vi "Configure Serial Bus (UART - Basic).vi"(0 "VISA resource name":refnum<visa-resource-name>, 1 "Bit Order (0: LSB First)":i32(ring) items=["LSB First", "MSB First"], 2 "Parity (0: Even)":i32(ring) items=["Even", "Odd", "None"], 3 "Data Bits (5 bits)":i32=5, 5 "Serial Bus Name (1: Serial Bus 1)":i32(ring)=1 items=["Serial Bus 1"=1, "Serial Bus 2"=2], 7 "Decode Base (2: Hex)":i32(ring)=2 items=["ASCII", "Binary", "Hex"], 9 "Baud Rate (9600 bps)":dbl=9600.0, 11 "error in (no error)":errorcluster, 12 "Packet Terminate Byte (-1)":i32=-1, 13 "Polarity (0: High)":i32(ring) items=["High", "Low"]) -> (4 "VISA resource name out":refnum<visa-resource-name>, 15 "error out":errorcluster)   [LabVIEW 2017, in "Agilent 2000 3000 X-Series.lvlib"]
doc: "Configures the basic settings of UART bus."
uses:
  Agilent 2000 3000 X-Series.lvlib
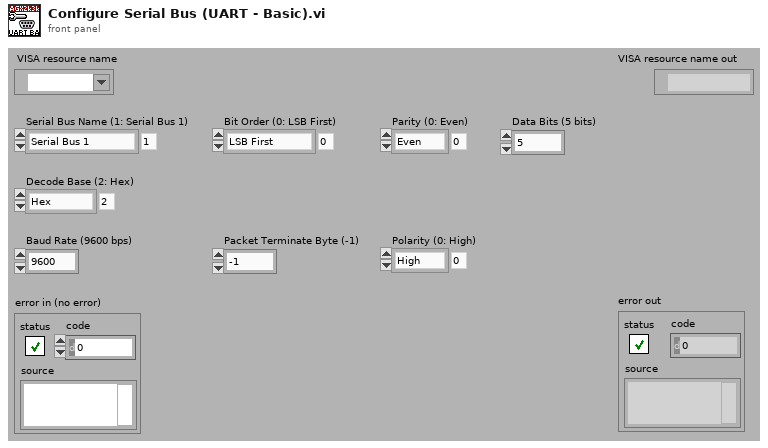
[diagram p1: front panel]
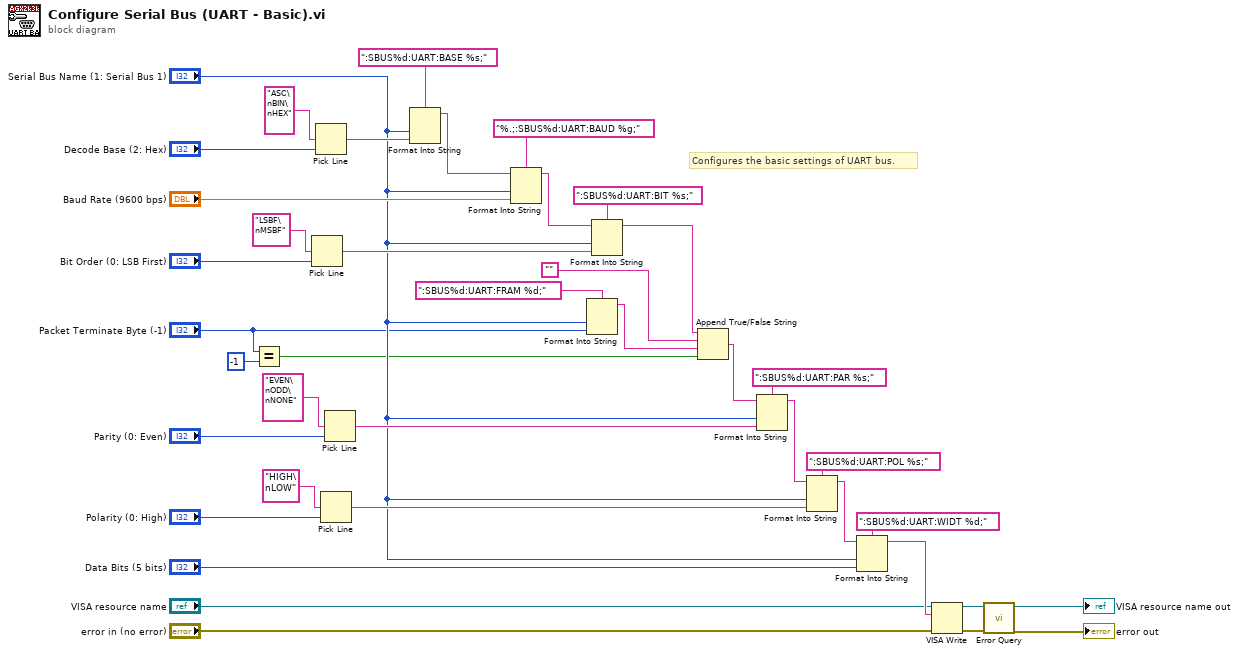
[diagram p0: block diagram]
diagram:
  # "Configures the basic settings of UART bus."
  n1 = Equal?(x="Packet Terminate Byte (-1)", y=-1 ("Packet Terminate Byte (-1)")) -> (x = y?=w5:bool)
  n2 = Pick Line(multi-line string="LSBF\nMSBF", line index="Bit Order (0: LSB First)") -> (output string=w29:string)  [unwired: 1 out]
  n3 = Pick Line(multi-line string="ASC\nBIN\nHEX", line index="Decode Base (2: Hex)") -> (output string=w37:string)  [unwired: 1 out]
  n4 = Pick Line(multi-line string="HIGH\nLOW", line index="Polarity (0: High)") -> (output string=w19:string)  [unwired: 1 out]
  n5 = Pick Line(multi-line string="EVEN\nODD\nNONE", line index="Parity (0: Even)") -> (output string=w24:string)  [unwired: 1 out]
  n6 = Format Into String(format string=":SBUS%d:UART:BASE %s;", "Serial Bus Name (1: Serial Bus 1)", w37) -> (resulting string=w36:string)  [unwired: 2 in, 1 out]
  n7 = Format Into String(format string="%.;:SBUS%d:UART:BAUD %g;", initial string=w36, "Serial Bus Name (1: Serial Bus 1)", "Baud Rate (9600 bps)") -> (resulting string=w31:string)  [unwired: 1 in, 1 out]
  n8 = Format Into String(format string=":SBUS%d:UART:FRAM %d;", "Serial Bus Name (1: Serial Bus 1)", "Packet Terminate Byte (-1)") -> (resulting string=w1:string)  [unwired: 2 in, 1 out]
  n9 = Format Into String(format string=":SBUS%d:UART:BIT %s;", initial string=w31, "Serial Bus Name (1: Serial Bus 1)", w29) -> (resulting string=w4:string)  [unwired: 1 in, 1 out]
  n10 = Append True/False String(1:w5, 2:w1, 3:"", 4:w4) -> (0:w3:string)
  n11 = Format Into String(format string=":SBUS%d:UART:PAR %s;", initial string=w3, "Serial Bus Name (1: Serial Bus 1)", w24) -> (resulting string=w21:string)  [unwired: 1 in, 1 out]
  n12 = Format Into String(format string=":SBUS%d:UART:POL %s;", initial string=w21, "Serial Bus Name (1: Serial Bus 1)", w19) -> (resulting string=w18:string)  [unwired: 1 in, 1 out]
  n13 = Format Into String(format string=":SBUS%d:UART:WIDT %d;", initial string=w18, "Serial Bus Name (1: Serial Bus 1)", "Data Bits (5 bits)") -> (resulting string=w15:string)  [unwired: 1 in, 1 out]
  n14 = VISA Write(VISA resource name="VISA resource name", write buffer=w15, error in (no error)="error in (no error)") -> (VISA resource name out=w12:refnum<visa-resource-name>, error out=w11:errorcluster)  [unwired: 1 out]
  n15 = call "Error Query.vi"("error in (no error)"=w11, "VISA resource name"=w12) -> ("error out"=→"error out":errorcluster, "VISA resource name out"=→"VISA resource name out":refnum<visa-resource-name>)  [unwired: 8 out]
